vi "AssertsNotEqual.vi"(0 "VI Reference In":refnum<vi>, 1 "Label (VI Title)":string="Default", 11 "error in (no error)":errorcluster) -> (4 "VI Reference Out":refnum<vi>, 15 "error out":errorcluster)   [LabVIEW 2016, in "Drona Test.lvlib"]
uses:
  Drona Test.lvlib
  main/apis/Stimulus/KeyBoardSimulation/ValueSignalLatchBooleanString.vi
  main/apis/Assert/AssertControlValue/NotEqual.vi
  <vilib>/addons/_JKI Toolkits/Caraya/classes/Assert/Assert Not Error.vi
  <vilib>/addons/_JKI Toolkits/Caraya/classes/Assert/Assert Error.vi
  <vilib>/addons/_JKI Toolkits/Caraya/classes/Test/Test.lvclass
  main/Drona.lvlib
  <vilib>/addons/_JKI Toolkits/Caraya/classes/Assert/Assert.lvclass
  main/apis/Stimulus/KeyBoardSimulation/KeyboardSimulation.lvlib
  main/apis/Assert/AssertControlValue/AssertControlValue.lvlib
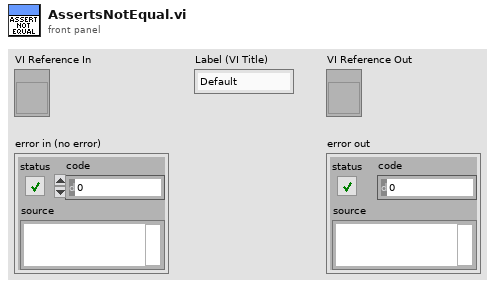
[diagram p1: front panel]
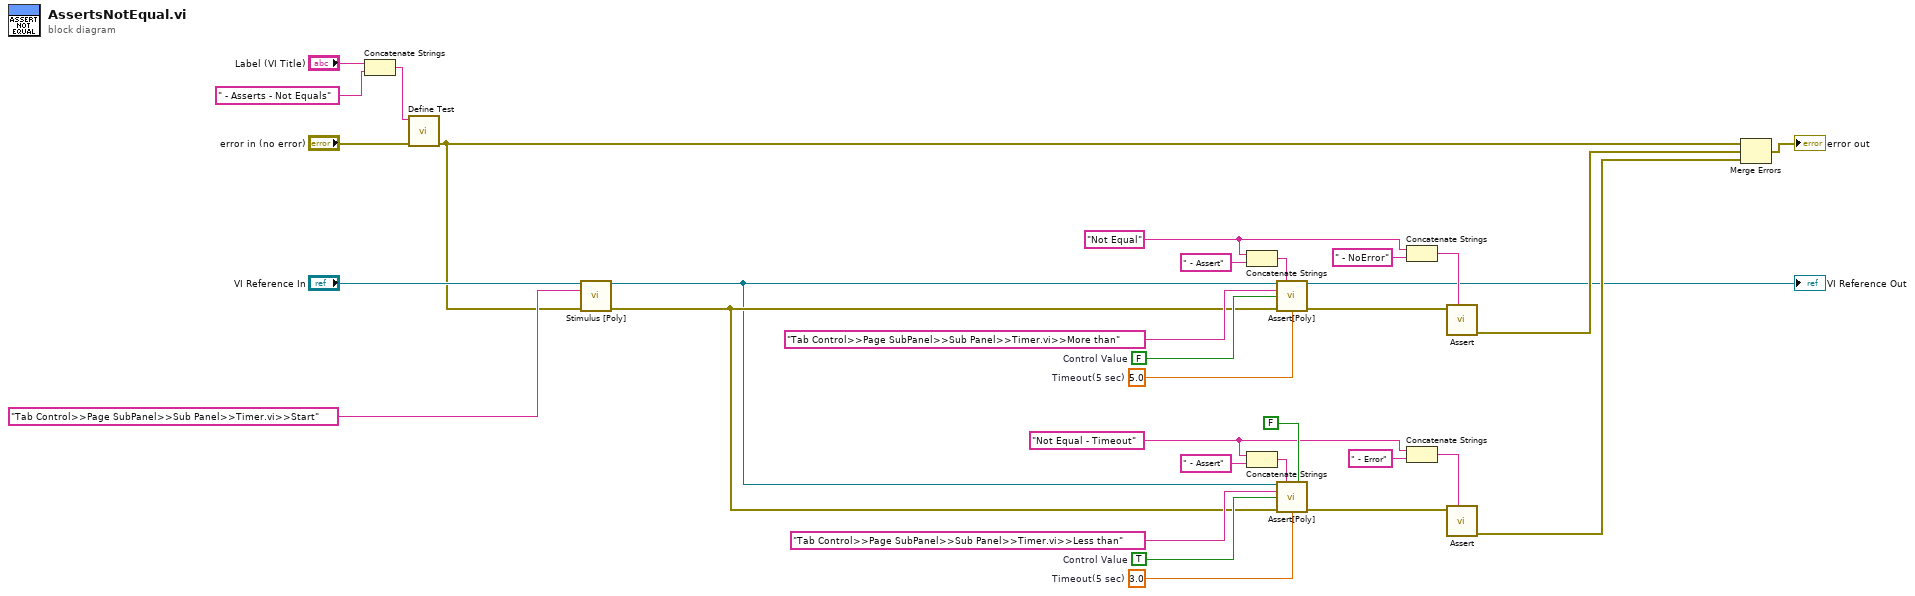
[diagram p0: block diagram]
diagram:
  w4 = TRUE  # Control Value
  w16 = 3.0  # Timeout(5 sec)
  w17 = "Not Equal - Timeout" ("string")
  w15 = 5.0  # Timeout(5 sec)
  w14 = FALSE  # Control Value
  w13 = "Not Equal" ("string")
  n1 = Concatenate Strings("Label (VI Title)", " - Asserts - Not Equals" ("Label (VI Title)")) -> (w28:string)
  n2 = call <vilib>:"Define Test.vi"("error in (no error)"="error in (no error)", "Label (VI Title)"=w28) -> ("error out"=w25:errorcluster)  [unwired: 9 in]
  n3 = call-poly "Stimulus [Poly].vi"("VI Reference In"="VI Reference In", "Control Path"="Tab Control>>Page SubPanel>>Sub Panel>>Timer.vi>>Start", "error in"=w25) -> ("VI Reference Out"=w2:refnum<vi>, "error out"=w3:errorcluster)  [unwired: 11 in]
  n4 = Concatenate Strings(w13, " - Assert" ("string")) -> (w11:string)
  n5 = Concatenate Strings(w17, " - Assert" ("string")) -> (w19:string)
  n6 = call-poly "Assert[Poly].vi"("VI Reference In"=w2, "Label"=w11, "Control Path"="Tab Control>>Page SubPanel>>Sub Panel>>Timer.vi>>More than", "Control Value"=w14, "Error In"=w3, "Timeout(5 sec)"=w15) -> ("VI Reference Out"=→"VI Reference Out":refnum<vi>, "Error Out"=w10:errorcluster)  [unwired: 8 in]
  n7 = call-poly "Assert[Poly].vi"("VI Reference In"=w2, "Label"=w19, "Assert Only? (F)"=FALSE, "Control Path"="Tab Control>>Page SubPanel>>Sub Panel>>Timer.vi>>Less than", "Control Value"=w4, "Error In"=w3, "Timeout(5 sec)"=w16) -> ("Error Out"=w20:errorcluster)  [unwired: 7 in, 1 out]
  n8 = Concatenate Strings(w13, " - NoError" ("string")) -> (w12:string)
  n9 = Concatenate Strings(w17, " - Error" ("string")) -> (w18:string)
  n10 = call-poly <vilib>:"Assert.vi"("Label"=w12, "Not Error?"=w10) -> ("error out"=w6:errorcluster)  [unwired: 9 in]
  n11 = call-poly <vilib>:"Assert.vi"("Label"=w18, "Error?"=w20) -> ("error out"=w5:errorcluster)  [unwired: 9 in]
  n12 = Merge Errors(w25, w6, w5) -> (→"error out":errorcluster)
